vi "Set Initialization Data - Opener.vi"(8 "error in":errorcluster, 11 "Server Client in":refnum<class "Server Client.lvclass">) -> (0 "error out":errorcluster, 3 "Server Client out":refnum<class "Server Client.lvclass">)   [LabVIEW 2020]
doc: "Sets the initialization data of a statically linked subWorker."
uses:
  <vilib>/addons/_Workers/Library/Classes/Worker/Worker.lvclass
  Opener/Initialization Data.ctl
  Opener/Opener.lvclass
  Server Client.lvclass
  C:/Program Files (x86)/National Instruments/LabVIEW 2020/vi.lib/addons/_Workers/Library/Classes/Worker User/Worker User.lvclass
  C:/Program Files (x86)/National Instruments/LabVIEW 2020/vi.lib/addons/_Workers/Library/Classes/Worker/Worker.lvclass
  C:/Program Files (x86)/National Instruments/LabVIEW 2020/vi.lib/addons/_Workers/Library/Classes/Workers Object/Workers Object.lvclass
  C:/Users/TestAdmin/git/TCP-Workers/Workers/Server Client/Server Client.lvclass
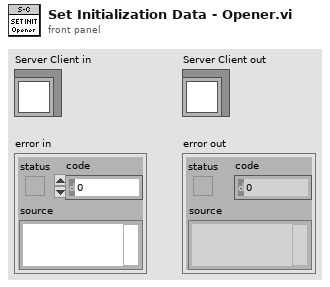
[diagram p1: front panel]
types:
  T1 = typedef "Opener.lvclass/Initialization Data.ctl" = cluster{"String":string}
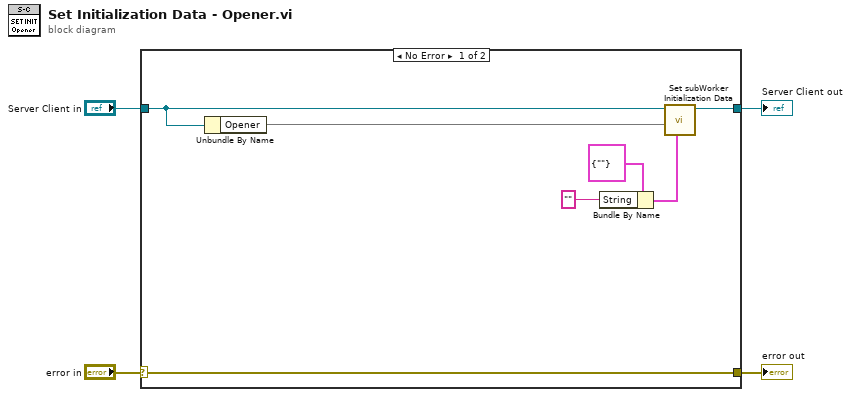
[diagram p0: block diagram]
diagram:
  n1 = case shown="No Error" "error in" {
    selector: "error in" -> [w11 w13]
    tunnel: [w11 w13] -> w3
    tunnel: [w9 w12] -> w2
    tunnel: "Server Client in" -> [w8 w12]
    frame No Error {
      n2 = Unbundle By Name(w8) -> ("Opener"=w10)
      n3 = Bundle By Name(cluster=T1 {"String"=""} ("Initialization Data"), "String"="" ("Placeholder")) -> (w6:T1)
      n4 = call <vilib>:"Set subWorker Initialization Data.vi"("Initialization Data"=w6, "subWorker"=w10, "Worker"=w8) -> ("Worker out"=w9:refnum<class "Server Client.lvclass">)  [unwired: 8 in]
    }
    frame Error {
    }
  }
  "error out" <- w3
  "Server Client out" <- w2
